vi "Class DVR API Generator.vi"() -> ()   [LabVIEW 2016]
uses:
  <vilib>/Utility/error.llb/DialogType.ctl
  Source/SLL Queued State Machine/Queue Driver/Create Queue.vi
  Source/SLL Queued State Machine/Queue Driver/Enqueue an Item to Queue.vi
  Source/SLL Queued State Machine/Queue Driver/Dequeue Queue.vi
  Source/SLL Queued State Machine/Queue Driver/Enqueue N Items.vi
  Source/SLL Queued State Machine/Queue Driver/Flush Queue.vi
  Source/SLL Queued State Machine/Queue Driver/Release Queue.vi
  Source/SLL Queued State Machine/SLL QSM.lvlib
  Source/SLL Scripting/SLL Scripting.lvlib
panel:
  out "Status":string
  in  "Run":bool
  in  "Method Folder Name":string="Methods"
  in  "DVR API Folder Name":string="APIs"
  in  "Class Path":path
  in  "DVR API Suffix":string=" API"
  # "Class DVR API Generator"
  # "Generates DVR based APIs for the class methods. \n\nSpecify the \n1. Class path, \n2. Methods folder where the class methods are present,\n3. DVR API folder where the DVR APIs needs to be created,\n4. Suffix for the DVR APIs to be generated"
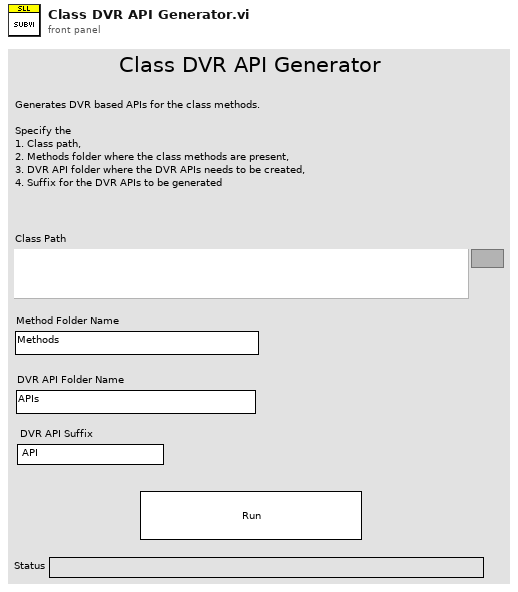
[diagram p1: front panel]
types:
  T1 = typedef "DialogType.ctl" = u16
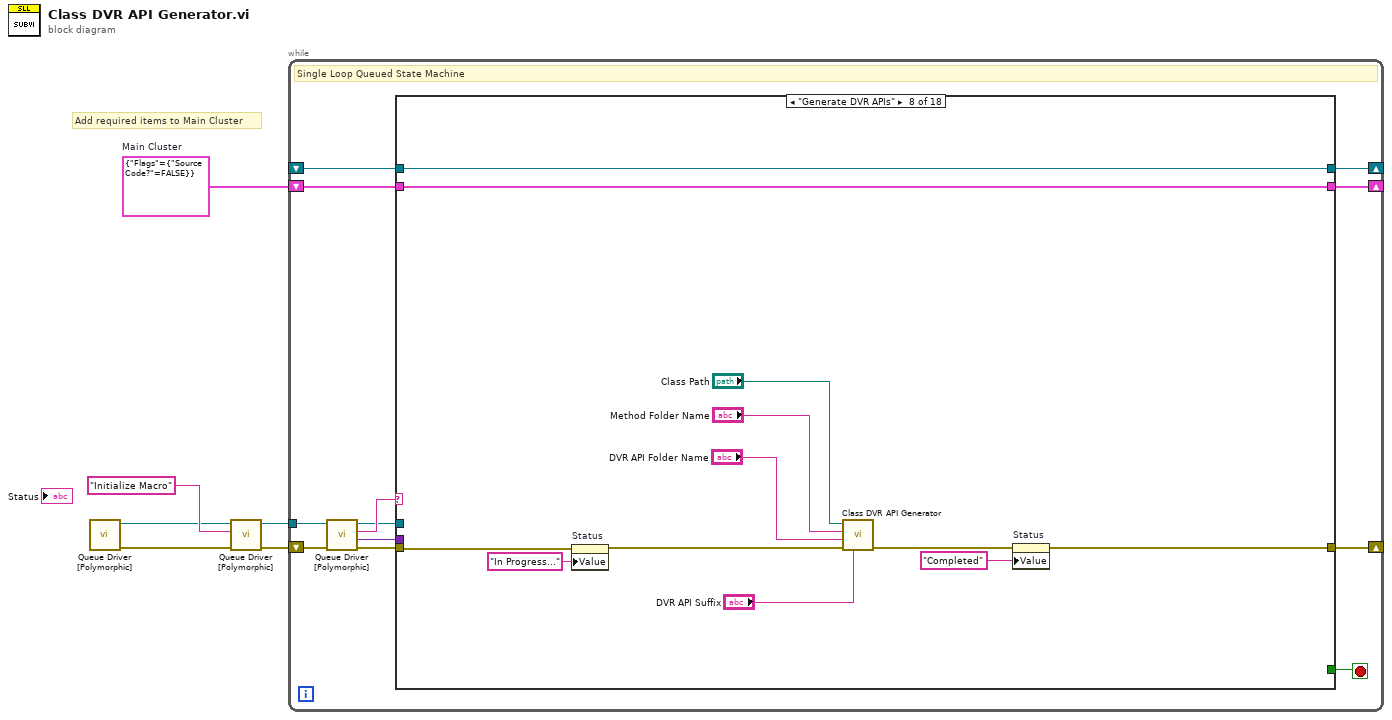
[diagram p0: block diagram]
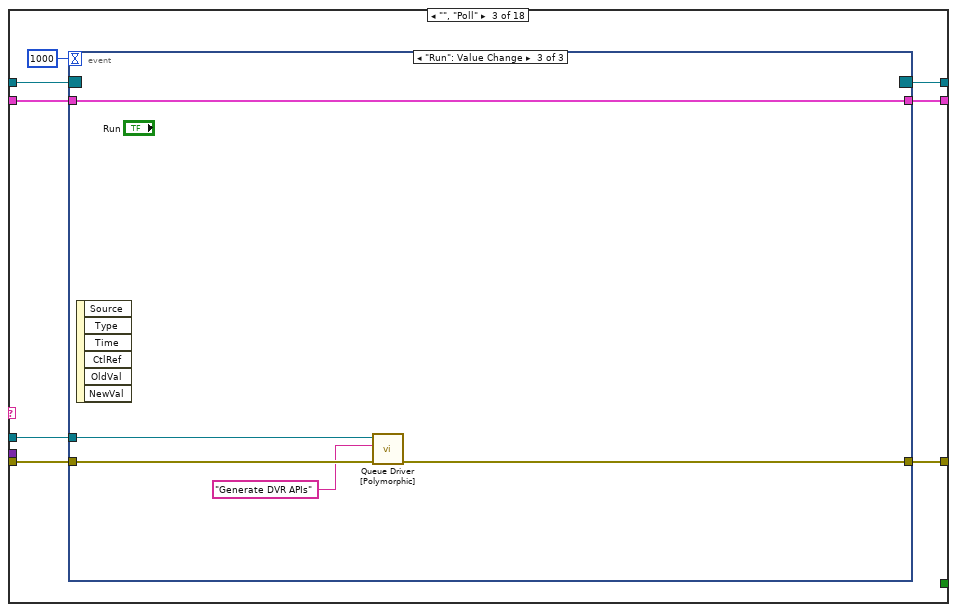
[diagram p4: hidden frame]
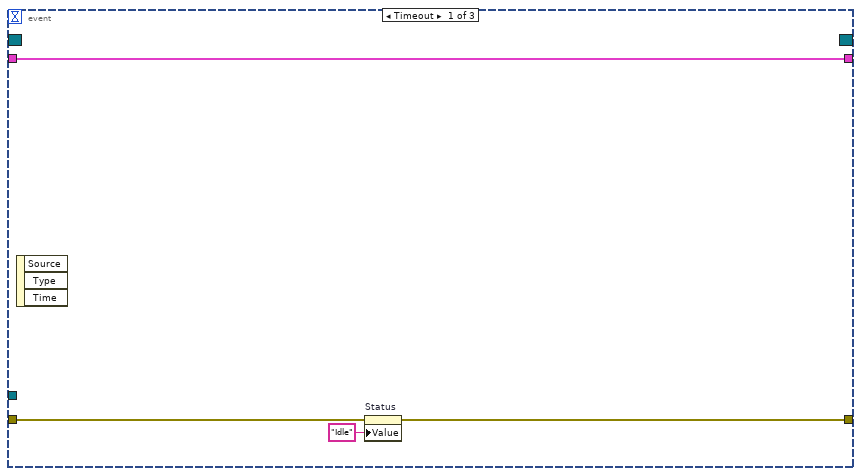
[diagram p5: hidden frame]
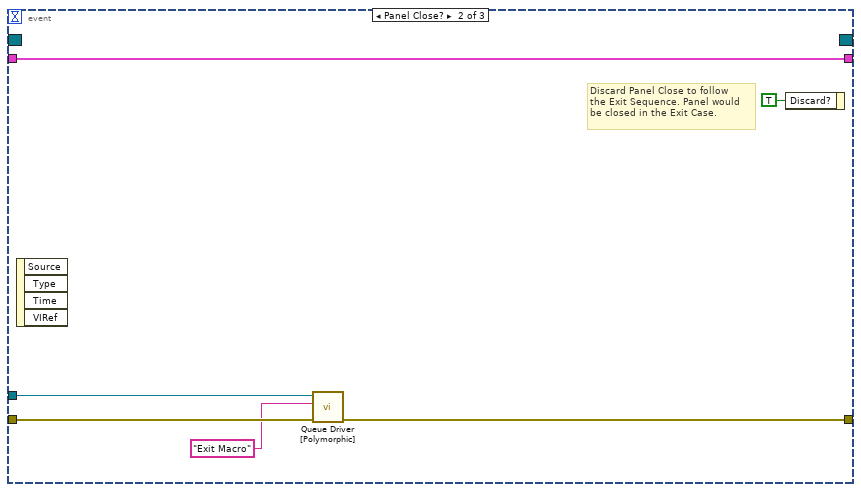
[diagram p6: hidden frame]
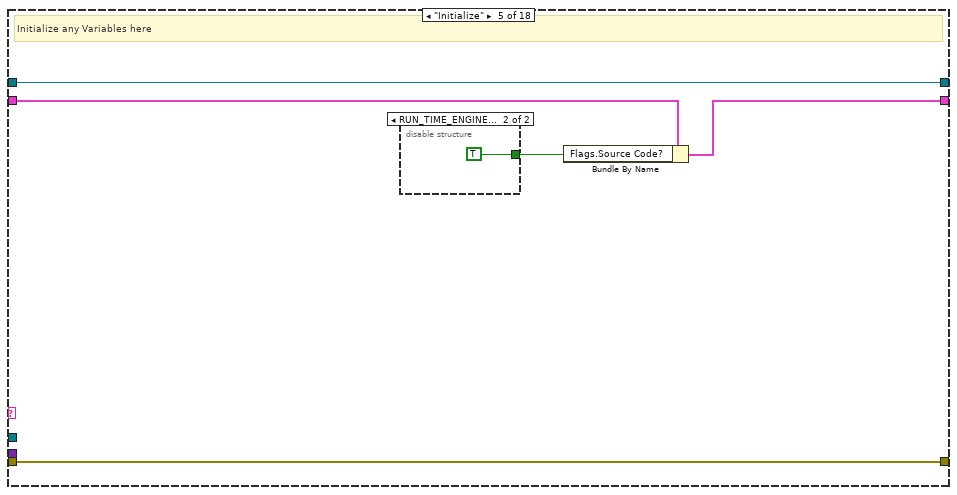
[diagram p8: hidden frame]
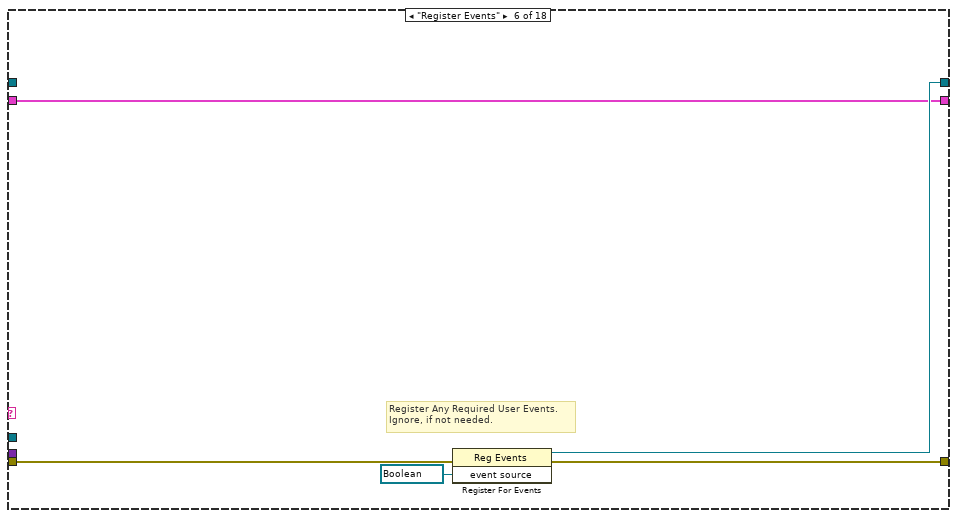
[diagram p10: hidden frame]
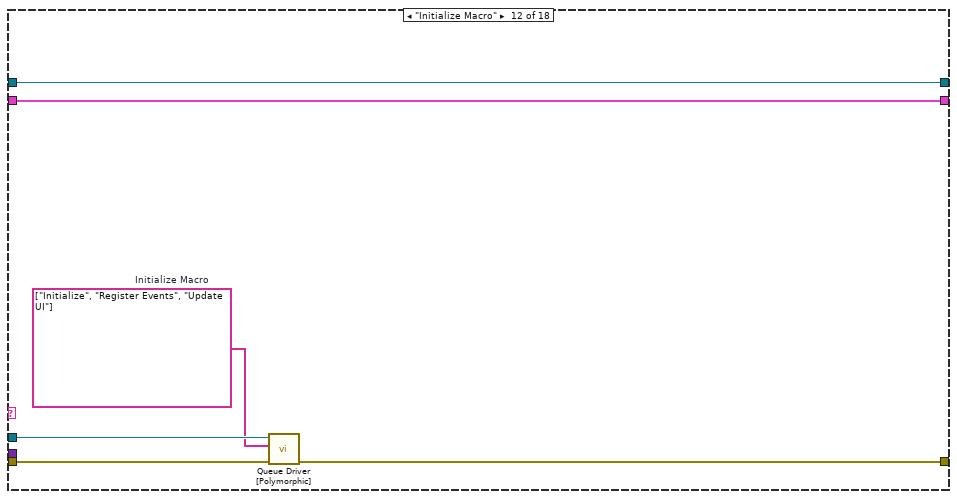
[diagram p15: hidden frame]
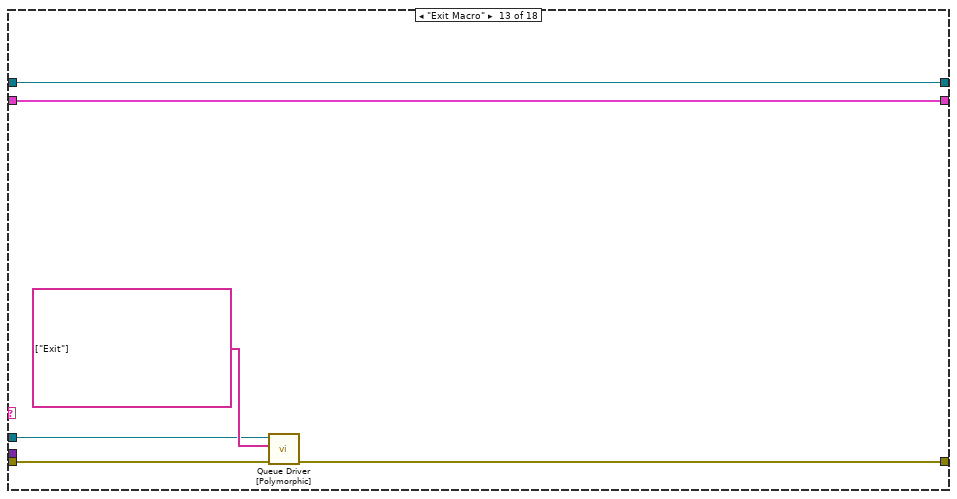
[diagram p16: hidden frame]
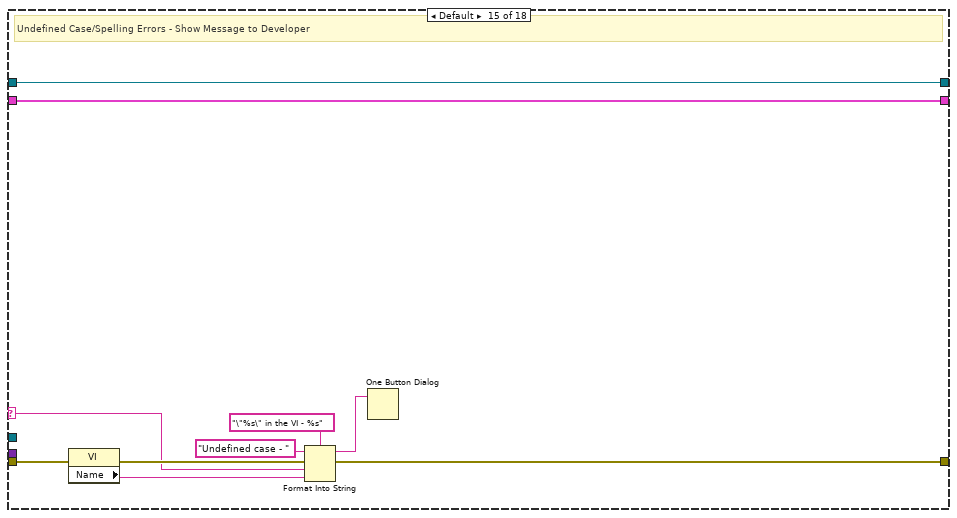
[diagram p18: hidden frame]
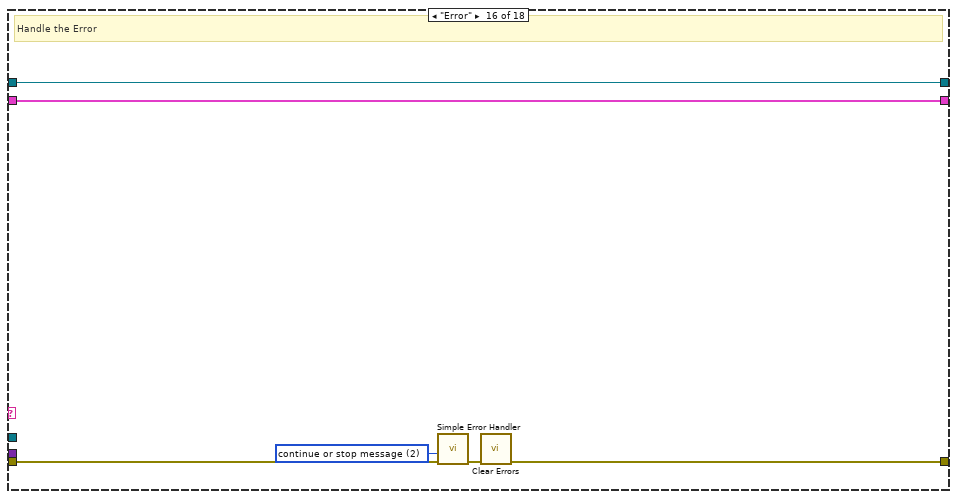
[diagram p19: hidden frame]
diagram:
  w4 = cluster{"Flags":cluster{"Source Code?":bool}} {"Flags"={"Source Code?"=FALSE}}  # Main Cluster
  # "Add required items to Main Cluster"
  n1 = call-poly "Queue Driver [Polymorphic].vi"() -> ("Error Out"=w6:errorcluster, "Queue Ref"=w2:refnum<queue>)  [unwired: 10 in]
  n2 = call-poly "Queue Driver [Polymorphic].vi"("Error In"=w6, "Item to Add"="Initialize Macro", "Queue Ref In"=w2) -> ("Error Out"=w5:errorcluster, "Queue Ref Out"=w1:refnum<queue>)  [unwired: 7 in]
  n3 = while "SLL Queued State Machine" {
    shift-right: [w16] -> _
    shift-left: w5 -> [w18]
    shift-right: [w14] -> _
    shift-left: _ -> [w13]
    shift-right: [w12] -> _
    shift-left: w4 -> [w11]
    tunnel: w1 -> [w9]
    stop <- w15 stop-if-true
    # "Single Loop Queued State Machine"
    n4 = call-poly "Queue Driver [Polymorphic].vi"("Error In"=w18, "Queue Ref In"=w9) -> ("Error Out"=w17:errorcluster, "Data"=w7:variant, "Dequeue"=w10:string, "Queue Ref Out"=w8:refnum<queue>)  [unwired: 6 in]
    n5 = case "QSM Case Structure" shown="\"Generate DVR APIs\"" w10 {
      selector: w10 -> [_ _ _ _ _ _ _ _ _ _ _ _ _ _ w101 _ _ _]
      tunnel: w17 -> [w21 w24 w30 w50 w55 w61 w64 w69 w79 w82 w85 w89 w95 w100 w104 w116 w119 w132]
      tunnel: [w21 w24 w31 w50 w55 w60 w64 w66 w79 w82 w85 w88 w94 w100 w107 w114 w119 w128] -> w16
      tunnel: [_ _ _ _ _ _ _ _ _ _ _ _ _ _ _ _ _ TRUE] -> w15
      tunnel: [w20 w23 w29 w49 w54 w59 w63 w76 w78 w81 w84 w91 w97 w99 w110 w113 w118 w131] -> w14
      tunnel: w13 -> [w20 w23 w28 w49 w54 _ w63 w76 w78 w81 w84 w91 w97 w99 w110 w113 w118 w131]
      tunnel: [w19 w22 w26 w48 w51 w58 w62 w75 w77 w80 w83 w90 w96 w98 w109 w112 w117 w130] -> w12
      tunnel: w11 -> [w19 w22 w27 w48 w52 w58 w62 w75 w77 w80 w83 w90 w96 w98 w109 w112 w117 w130]
      tunnel: w8 -> [_ _ w25 _ _ _ _ _ _ _ _ w87 w92 _ _ _ _ w121]
      tunnel: w7 -> [_ _ _ _ _ _ _ _ _ _ _ _ _ _ _ _ _ _]
      frame "/--------------- Read Me -----------------/" {
        # "General Purpose Queue Based State Machine for Any Use Case (main application, module, pop up message etc)\n\nAdvantages:\n1. No Need to Pass Queue References between Queue Driver VIs.\n2. This template can be safely used in multiple parallel running modules without any issues.\n3. This template can also be safely used even in cases where the VI is configured to be a Clone, where multiple \ninstances of the VI could be executing concurrently.\n\nHow to Use:\n1. Add necessary items to the Main Cluster.\n2. Use the Polymorphic Queue Driver for doing any queue operations. There is no need to pass the queue driver\nreference, as the Queue Driver automatically infers the reference based on the VI instance from which it is called.\n3. Add any required user events in the \"Register Events\" case. Ignore if not needed.\n4. Use \"Sequences\" section for defining any list of state calls, which could be used in multiple places. \nEg: Initialize Sequence, might be needed if we need to any reinitialization."
      }
      frame "/------------------ Poll -------------------/" {
      }
      frame "", "Poll" {
        n6 = event shown="[2] \"Run\": Value Change" {
          selector: w28 -> [_ _ _]
          dyn-events: [_ _ _] -> w29
          timeout: 1000 -> [_ _ _]
          tunnel: [w33 w41 w46] -> w31
          tunnel: w30 -> [w34 w42 w47]
          tunnel: w27 -> [w36 w40 w45]
          tunnel: [w36 w40 w45] -> w26
          tunnel: w25 -> [_ w37 w43]
          event Timeout {
            n7 = event-data() -> ()  [unwired: 1 in, 3 out]
            n8 = property on="Status" class="Str"(error in=w34, "Value"="Idle" ("Status")) -> (error out=w33:errorcluster)  [unwired: 1 in, 1 out]
          }
          event Panel Close? {
            # "Discard Panel Close to follow\nthe Exit Sequence. Panel would\nbe closed in the Exit Case."
            n9 = event-data() -> ()  [unwired: 1 in, 4 out]
            n10 = call-poly "Queue Driver [Polymorphic].vi"("Error In"=w42, "Item to Add"="Exit Macro" ("Enqueue"), "Queue Ref In"=w37) -> ("Error Out"=w41:errorcluster)  [unwired: 7 in, 1 out]
            n11 = event-data("Discard?"=TRUE) -> ()  [unwired: 1 in, 1 out]
          }
          event "Run": Value Change {
            n12 = event-data() -> ()  [unwired: 1 in, 6 out]
            n13 = call-poly "Queue Driver [Polymorphic].vi"("Error In"=w47, "Item to Add"="Generate DVR APIs" ("Enqueue"), "Queue Ref In"=w43) -> ("Error Out"=w46:errorcluster)  [unwired: 7 in, 1 out]
          }
        }
      }
      frame "/--------------- Initialize -----------------/" {
      }
      frame "Initialize" {
        # "Initialize any Variables here"
        n14 = disable-structure shown="RUN_TIME_ENGINE==False" {
          disable-tunnel: [_ TRUE] -> w53
          frame condition #0 {
          }
          frame condition #1 (active) {
          }
        }
        n15 = Bundle By Name(cluster=w52, "Flags.Source Code?"=w53) -> (w51:cluster{"Flags":cluster{"Source Code?":bool}})
      }
      frame "Register Events" {
        # "Register Any Required User Events. \nIgnore, if not needed."
        n16 = register-events(error in=w61, refnum<vi> refnum ("event source")) -> (reference out=w59:refnum<event-registration>, error out=w60:errorcluster)  [unwired: 1 in]
      }
      frame "/---------- Custom Case Splitter ----------/" {
      }
      frame "Generate DVR APIs" {
        n17 = property on="Status" class="Str"(error in=w69, "Value"="In Progress..." ("Status")) -> (error out=w70:errorcluster)  [unwired: 1 in, 1 out]
        n18 = call "Class DVR API Generator.vi"("DVR API Suffix"="DVR API Suffix", "error in (no error)"=w70, "DVR API Folder Name"="DVR API Folder Name", "Method Folder Name"="Method Folder Name", "Class Path"="Class Path") -> ("error out"=w67:errorcluster)  [unwired: 6 in]
        n19 = property on="Status" class="Str"(error in=w67, "Value"="Completed" ("Status")) -> (error out=w66:errorcluster)  [unwired: 1 in, 1 out]
      }
      frame "/-------------- User Interface --------------/" {
        # "Duplicate this case to create additional case splitters for readability"
      }
      frame "Update UI" {
        # "Update Front Panel Controls in this Case"
      }
      frame "/----------------- Macros -----------------/" {
      }
      frame "Initialize Macro" {
        w86 = string[] ["Initialize", "Register Events", "Update UI"]  # Initialize Macro
        n20 = call-poly "Queue Driver [Polymorphic].vi"("Error In"=w89, "Enqueue N"=w86, "Queue Ref In"=w87) -> ("Error Out"=w88:errorcluster)  [unwired: 7 in, 1 out]
      }
      frame "Exit Macro" {
        n21 = call-poly "Queue Driver [Polymorphic].vi"("Error In"=w95, "Enqueue N"=string[] ["Exit"], "Queue Ref In"=w92) -> ("Error Out"=w94:errorcluster)  [unwired: 7 in, 1 out]
      }
      frame "/-------------- Error Handler--------------/" {
      }
      frame Default {
        # "Undefined Case/Spelling Errors - Show Message to Developer"
        n22 = property class="VI"(error in=w104) -> (error out=w103:errorcluster, "Name"=w102:string)  [unwired: 1 in, 1 out]
        n23 = Format Into String(format string="\"%s\" in the VI - %s" ("message"), initial string="Undefined case - ", error in=w103, w101, w102) -> (resulting string=w105:string, error out=w107:errorcluster)
        n24 = One Button Dialog(message=w105) -> ()  [unwired: 1 in, 1 out]
      }
      frame "Error" {
        w111 = T1 2 items=["no dialog", "OK message", "continue or stop message", "OK message + warnings", "continue/stop + warnings"] ("type of dialog (OK msg:1)")
        # "Handle the Error"
        n25 = call <vilib>:"Simple Error Handler.vi"("type of dialog (OK msg:1)"=w111, "error in (no error)"=w116) -> ("error out"=w115:errorcluster)  [unwired: 3 in, 4 out]
        n26 = call <vilib>:"Clear Errors.vi"("error in (no error)"=w115) -> ("error out"=w114:errorcluster)  [unwired: 5 in, 1 out]
      }
      frame "/------------------- Exit --------------------/" {
      }
      frame "Exit" {
        n27 = call-poly "Queue Driver [Polymorphic].vi"("Error In"=w132, "Queue Ref In"=w121) -> ("Error Out"=w133:errorcluster, "Queue Ref Out"=w120:refnum<queue>)  [unwired: 7 in, 1 out]
        n28 = Unbundle By Name(w130) -> ("Flags.Source Code?"=w123:bool)
        n29 = call-poly "Queue Driver [Polymorphic].vi"("Error In"=w133, "Queue Ref In"=w120) -> ("Error Out"=w129:errorcluster)  [unwired: 9 in]
        n30 = Call Chain() -> (call chain=w127:string[])
        n31 = Array Size(array=w127) -> (size(s)=w126:i32)
        n32 = Equal?(x=w126, y=1) -> (x = y?=w124:bool)
        n33 = And(x=w123, y=w124) -> (x .and. y?=w122:bool)
        n34 = case "Skip Panel Close when in Source\nCode and is the top most caller" shown="True" w122 {
          tunnel: w129 -> [w136 w138]
          tunnel: [w137 w138] -> w128
          frame False {
            # "Close Panel"
            n35 = invoke class="VI" method="FP.Close"() -> (error out=w135:errorcluster)  [unwired: 3 in, 2 out]
            n36 = Merge Errors(w136, w135) -> (w137:errorcluster)
          }
          frame True {
            # "Do Not Close Panel"
          }
        }
      }
    }
  }
